vi "TimerPGM to String.vi"(8 "error in":errorcluster, 9 "Step No.":i32, 10 "PGM No.":i32, 11 "Op./Stop Mode":T1) -> (0 "error out":errorcluster, 3 "String out":string)   [LabVIEW 2021, in "Environment Chamber.lvlib" / "Climatic Chamber.lvlib"]
uses:
  Climatic Chamber.lvlib
  Type Defs/Operation_Stop Mode Enum.ctl
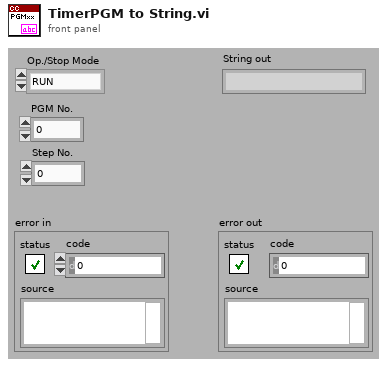
[diagram p1: front panel]
types:
  T1 = typedef "Environment Chamber.lvlib/Climatic Chamber.lvlib/Operation_Stop Mode Enum.ctl" = enum16{"RUN", "CONSTANT", "STANDBY", "OFF"}
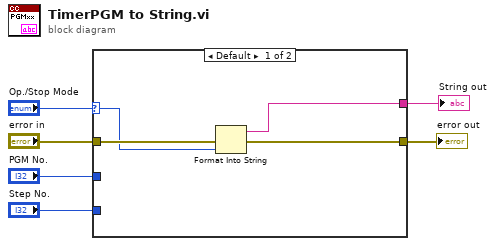
[diagram p0: block diagram]
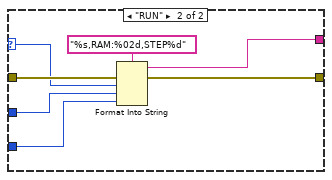
[diagram p2: hidden frame]
diagram:
  n1 = case shown="Default" "Op./Stop Mode" {
    selector: "Op./Stop Mode" -> [w8 w15]
    tunnel: "error in" -> [w10 w16]
    tunnel: [w9 w14] -> w5
    tunnel: "PGM No." -> [_ w13]
    tunnel: "Step No." -> [_ w12]
    tunnel: [w7 w11] -> w1
    frame Default {
      n2 = Format Into String(error in=w10, w8) -> (resulting string=w7:string, error out=w9:errorcluster)  [unwired: 2 in]
    }
    frame "RUN" {
      n3 = Format Into String(format string="%s,RAM:%02d,STEP%d", error in=w16, w15, w13, w12) -> (resulting string=w11:string, error out=w14:errorcluster)  [unwired: 1 in]
    }
  }
  "error out" <- w5
  "String out" <- w1
